vi "0037-Sub_map_backup.vi"() -> ()   [LabVIEW 2014]
uses:
  LVProject/private/CP2112_device.ctl
  LVProject/private/CP2112_SMBUS_S0.ctl
panel:
  out "配列":bool[](array[boolean])
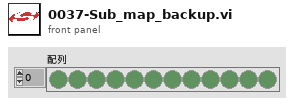
[diagram p1: front panel]
types:
  T1 = typedef "CP2112_device.ctl" = i32
  T2 = typedef "CP2112_SMBUS_S0.ctl" = enum8{"HID_SMBUS_S0_IDLE", "HID_SMBUS_S0_BUSY", "HID_SMBUS_S0_COMPLETE", "HID_SMBUS_S0_ERROR"}
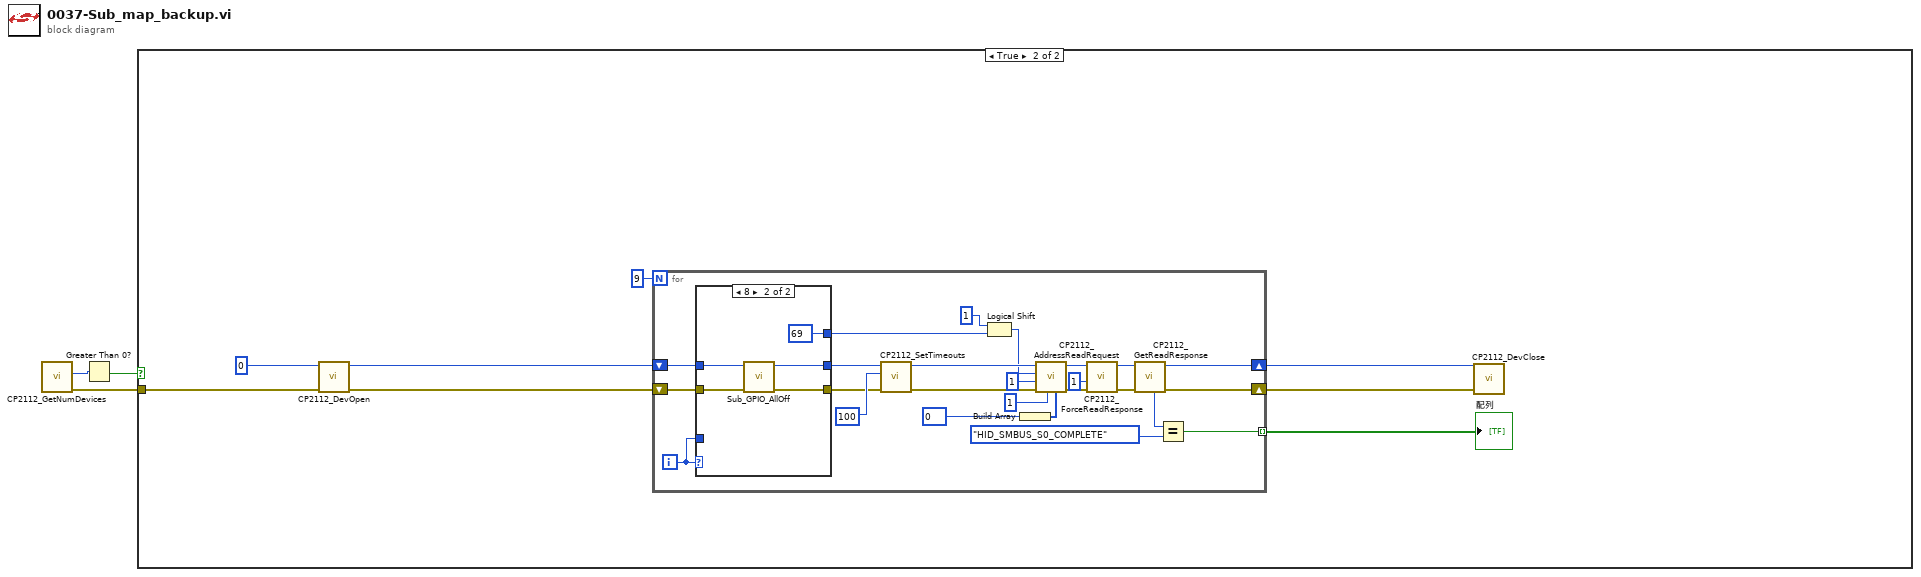
[diagram p0: block diagram]
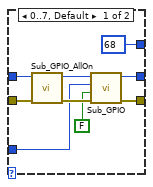
[diagram p3: hidden frame]
diagram:
  n1 = call "CP2112_GetNumDevices.vi"() -> ("error out"=w3:errorcluster, "numDevices"=w1:i32)  [unwired: 9 in, 1 out]
  n2 = Greater Than 0?(x=w1) -> (x > 0?=w2:bool)
  n3 = case shown="TRUE" w2 {
    tunnel: w3 -> [_ w10]
    frame False {
    }
    frame True {
      n4 = call "CP2112_DevOpen.vi"("error in (no error)"=w10, "deviceNum"=T1 0 ("device")) -> ("error out"=w9:errorcluster, "device"=w8:T1)  [unwired: 7 in, 1 out]
      n5 = for {
        N: 9 -> [_]
        shift-right: [w19] -> w6
        shift-left: w9 -> [w16]
        shift-right: [w20] -> w7
        shift-left: w8 -> [w14]
        tunnel: [w18] -> w4 mode=indexing
        i -> [w12]
        n6 = case shown="8" w12 {
          tunnel: [68 ("x") 69 ("x")] -> w17
          tunnel: w16 -> [w44 w49]
          tunnel: [w41 w47] -> w15
          tunnel: w14 -> [w43 w48]
          tunnel: [w40 w46] -> w13
          tunnel: w12 -> [w37 _]
          frame 0..7, Default {
            n7 = call "Sub_GPIO_AllOn.vi"("エラー出力 2"=w44, "device"=w43) -> ("エラー出力"=w42:errorcluster, "deviceOut"=w39:T1)  [unwired: 8 in]
            n8 = call "Sub_GPIO.vi"("エラー出力 2"=w42, "ブール"=FALSE, "GPIO"=w37, "device"=w39) -> ("エラー出力"=w41:errorcluster, "deviceOut"=w40:T1)  [unwired: 6 in]
          }
          frame 8 {
            n9 = call "Sub_GPIO_AllOff.vi"("エラー出力 2"=w49, "device"=w48) -> ("エラー出力"=w47:errorcluster, "deviceOut"=w46:T1)  [unwired: 8 in]
          }
        }
        n10 = call "CP2112_SetTimeouts.vi"("error in (no error)"=w15, "responseTimeout"=u32 100, "device"=w13) -> ("error out"=w34:errorcluster, "deviceOut"=w35:T1)  [unwired: 6 in, 1 out]
        n11 = Logical Shift(y=1, x=w17) -> (x << y=w23:i32)
        n12 = Build Array(u8 0 ("targetAddressSize")) -> (w27:u8[])
        n13 = call "CP2112_AddressReadRequest.vi"("targetAddress[]"=w27, "targetAddressSize"=u8 1, "error in (no error)"=w34, "numByteToRead"=i16 1, "slaveAddress"=w23, "device"=w35) -> ("error out"=w32:errorcluster, "deviceOut"=w33:T1)  [unwired: 3 in, 1 out]
        n14 = call "CP2112_ForceReadResponse.vi"("error in (no error)"=w32, "numByteToRead"=i16 1, "device"=w33) -> ("error out"=w31:errorcluster, "deviceOut"=w30:T1)  [unwired: 6 in, 1 out]
        n15 = call "CP2112_GetReadResponse.vi"("error in (no error)"=w31, "device"=w30) -> ("error out"=w19:errorcluster, "deviceOut"=w20:T1, "HID_SMBUS_S0"=w21:T2)  [unwired: 4 in, 3 out]
        n16 = Equal?(x=w21, y=CP2112_SMBUS_S0."HID_SMBUS_S0_COMPLETE" ("HID_SMBUS_S0")) -> (x = y?=w18:bool)
      }
      "配列" <- w4
      n17 = call "CP2112_DevClose.vi"("error in (no error)"=w6, "device"=w7) -> ()  [unwired: 9 in, 1 out]
    }
  }
